vi "Init.vi"() -> (3 "TEMPLATE Actor out":refnum<class "TEMPLATE Actor.lvclass">)   [LabVIEW 2020, in "_Template.lvlib" / "Templates.lvlib" / "TEMPLATE Actor.lvlib" / "TEMPLATE Actor.lvclass"]
uses:
  TEMPLATE Actor.lvclass
  jettl/jettl/Actor/Actor/Actor.lvclass
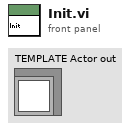
[diagram p1: front panel]
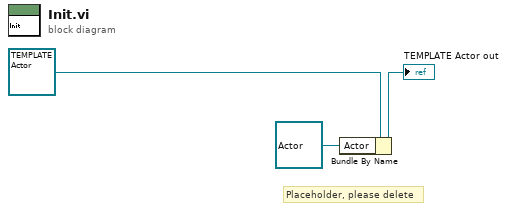
[diagram p0: block diagram]
diagram:
  # "Placeholder, please delete"
  n1 = Bundle By Name(cluster=refnum<class "TEMPLATE Actor.lvclass"> refnum ("TEMPLATE Actor out"), "Actor"=refnum<class "Actor.lvclass"> refnum) -> (→"TEMPLATE Actor out":refnum<class "TEMPLATE Actor.lvclass">)
